vi "Cache.SystemID.Fglb.vi"(5 "Station":string, 7 "Action (get)":T2=enum."get", 8 "error in (no error)":errorcluster, 10 "SytemID":T1, 11 "Variant":string) -> (0 "error out":errorcluster, 1 "Found":bool, 2 "SytemID":T1)   [LabVIEW 2016]
uses:
  Cache.SystemID.Fglb.Action.ctl
  Database/ProdaNG/Controls/ProdaNG.Identification.ctl
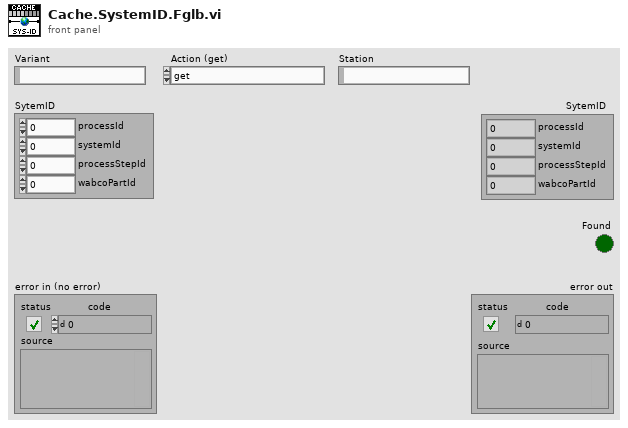
[diagram p1: front panel]
types:
  T1 = typedef "ProdaNG.Identification.ctl" = cluster{"processId":i32, "systemId":i32, "processStepId":i32, "wabcoPartId":i32}
  T2 = typedef "Cache.SystemID.Fglb.Action.ctl" = enum16{"init", "add", "get"}
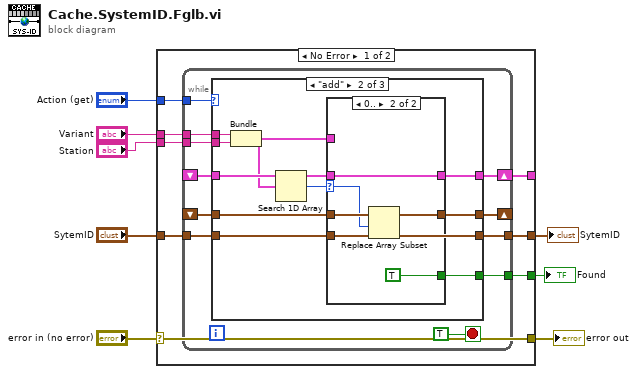
[diagram p0: block diagram]
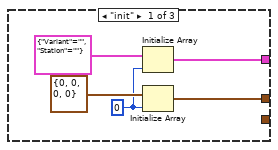
[diagram p2: hidden frame]
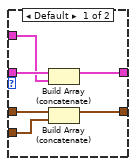
[diagram p3: hidden frame]
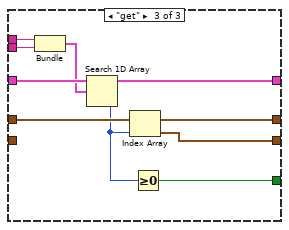
[diagram p4: hidden frame]
diagram:
  n1 = case shown="No Error" "error in (no error)" {
    selector: "error in (no error)" -> [w15 w63]
    tunnel: [w15 w63] -> w7
    tunnel: "SytemID" -> [w13 _]
    tunnel: "Action (get)" -> [w14 _]
    tunnel: "Variant" -> [w16 _]
    tunnel: [w12 _] -> _
    tunnel: [w11 _] -> w3
    tunnel: [w10 _] -> w2
    tunnel: "Station" -> [w9 _]
    frame No Error {
      n2 = while {
        tunnel: w16 -> [w24]
        tunnel: w14 -> [w27]
        shift-right: [w26] -> w12
        shift-left: _ -> [w25]
        shift-right: [w23] -> _
        shift-left: _ -> [w22]
        tunnel: w13 -> [w21]
        tunnel: [w19] -> w11
        tunnel: [w18] -> w10
        tunnel: w9 -> [w17]
        stop <- TRUE stop-if-true
        n3 = case shown="\"add\"" w27 {
          tunnel: [w28 w42 w62] -> w26
          tunnel: w25 -> [_ w35 w62]
          tunnel: w24 -> [_ w37 w59]
          tunnel: [w32 w41 w61] -> w23
          tunnel: w22 -> [_ w40 w61]
          tunnel: w21 -> [_ w33 _]
          tunnel: [_ w39 w60] -> w19
          tunnel: [_ w33 w55] -> w18
          tunnel: w17 -> [_ w36 w58]
          frame "init" {
            w29 = 0 ("dimension size")
            n4 = Initialize Array(cluster{"Variant":string, "Station":string} {"Variant"="", "Station"=""}, w29) -> (w28:cluster{"Variant":string, "Station":string}[])
            n5 = Initialize Array(T1 {"processId"=0, "systemId"=0, "processStepId"=0, "wabcoPartId"=0} ("Sytem"), w29) -> (w32:T1[])
          }
          frame "add" {
            n6 = Bundle("Variant"=w37, "Station"=w36) -> (w34:cluster{"Variant":string, "Station":string})  [unwired: 1 in]
            n7 = Search 1D Array(1D array=w35, element=w34) -> (index of element=w38:i32)  [unwired: 1 in]
            n8 = case shown="0.." w38 {
              selector: w38 -> [_ w51]
              tunnel: w35 -> [w48 w54]
              tunnel: w40 -> [w46 w53]
              tunnel: w34 -> [w44 _]
              tunnel: [w47 w54] -> w42
              tunnel: [w45 w52] -> w41
              tunnel: [_ TRUE] -> w39
              tunnel: w33 -> [w43 w49]
              frame Default {
                n9 = Build Array (concatenate)(w48, w44) -> (w47:cluster{"Variant":string, "Station":string}[])
                n10 = Build Array (concatenate)(w46, w43) -> (w45:T1[])
              }
              frame 0.. {
                n11 = Replace Array Subset(array=w53, new element=w49, index=w51) -> (w52:T1[])
              }
            }
          }
          frame "get" {
            n12 = Bundle("Variant"=w59, "Station"=w58) -> (w57:cluster{"Variant":string, "Station":string})  [unwired: 1 in]
            n13 = Search 1D Array(1D array=w62, element=w57) -> (index of element=w56:i32)  [unwired: 1 in]
            n14 = Index Array(array=w61, index=w56) -> (element=w55:T1)
            n15 = Greater Or Equal To 0?(x=w56) -> (x >= 0?=w60:bool)
          }
        }
      }
    }
    frame Error {
    }
  }
  "error out" <- w7
  "Found" <- w3
  "SytemID" <- w2
